vi "Periodic Tasks.vi"(8 "error in":errorcluster) -> ()   [LabVIEW 2020]
doc: "This VI runs in parallel to other robot code. It can contain as many user-defined periodic loops as you need. These can carry out PID or other sorts of timed response."
uses:
  <vilib>/Rock Robotics/Network Tables/NT Read Number.vi
  vi's/Global Variables.vi
  <vilib>/Rock Robotics/Network Tables/NT Read Numeric Array.vi
  <vilib>/Rock Robotics/Network Tables/NT Write Numeric Array.vi
  <vilib>/Rock Robotics/Network Tables/NT Write Number.vi
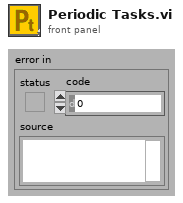
[diagram p1: front panel]
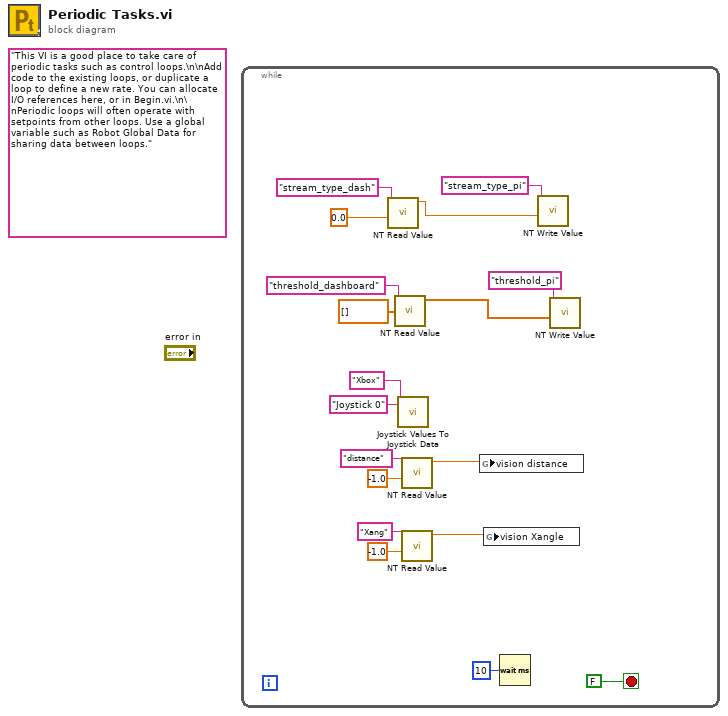
[diagram p0: block diagram]
diagram:
  (unwired) "This VI is a good place to take care of periodic tasks such as control loops.\n\nAdd code to the existing loops, or duplicate a loop to define a new rate. You can allocate I/O references here, or in Begin.vi.\n\nPeriodic loops will often operate with setpoints from other loops. Use a global variable such as Robot Global Data for sharing data between loops."
  n1 = while {
    stop <- FALSE stop-if-true
    n2 = call-poly <vilib>:"NT Read Value.vi"("Default Value"=0.0, "Name"="stream_type_dash") -> ("Numeric"=w4:dbl)  [unwired: 8 in, 1 out]
    n3 = call-poly <vilib>:"NT Read Value.vi"("Default Value"=dbl[] [], "Name"="threshold_dashboard") -> ("Numeric Array"=w7:dbl[])  [unwired: 8 in, 1 out]
    n4 = call "Joystick Values To Joystick Data.vi"("Xbox Name"="Xbox", "F310 Name"="Joystick 0" ("Xbox Name")) -> ()  [unwired: 18 in]
    n5 = call-poly <vilib>:"NT Read Value.vi"("Default Value"=-1.0, "Name"="distance") -> ("Numeric"=w13:dbl)  [unwired: 8 in, 1 out]
    n6 = call-poly <vilib>:"NT Read Value.vi"("Default Value"=-1.0, "Name"="Xang") -> ("Numeric"=w12:dbl)  [unwired: 8 in, 1 out]
    n7 = global write "Global Variables.vi" "vision distance"(w13) -> ()
    n8 = global write "Global Variables.vi" "vision Xangle"(w12) -> ()
    n9 = Wait (ms)(milliseconds to wait=u32 10) -> ()  [unwired: 1 out]
    n10 = call-poly <vilib>:"NT Write Value.vi"("Numeric"=w4, "Name"="stream_type_pi") -> ()  [unwired: 9 in, 1 out]
    n11 = call-poly <vilib>:"NT Write Value.vi"("Numeric Array"=w7, "Name"="threshold_pi") -> ()  [unwired: 9 in, 1 out]
  }
